vi "motor_outfeed_power.vi"(10 "Eject_Imp":dbl, 11 "Eject_Driver":dbl) -> (3 "Ele_Outfeed_Power_Power":dbl)   [LabVIEW 2014]
panel:
  in  "Outfeed Scalar [0,1]":dbl=1.0
  # "This is the motor outfeed power conversion"
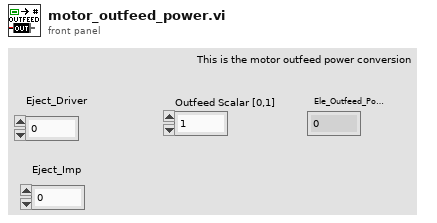
[diagram p1: front panel]
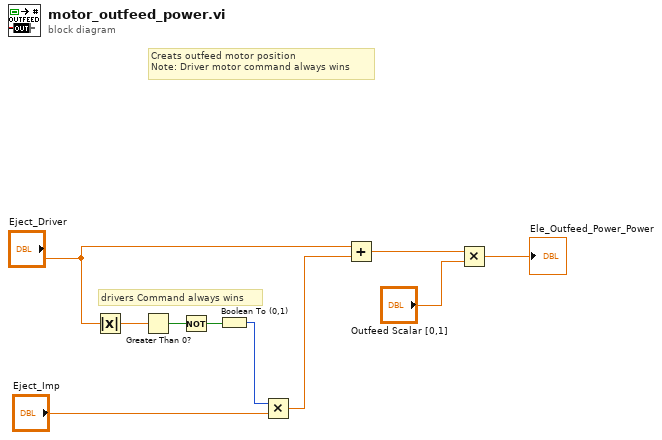
[diagram p0: block diagram]
diagram:
  # "drivers Command always wins"
  # "Creats outfeed motor position \nNote: Driver motor command always wins"
  n1 = Absolute Value(x="Eject_Driver") -> (abs(x)=w8:dbl)
  n2 = Greater Than 0?(x=w8) -> (x > 0?=w7:bool)
  n3 = Not(x=w7) -> (.not. x?=w5:bool)
  n4 = Boolean To (0,1)(Boolean=w5) -> (0, 1=w4:i16)
  n5 = Multiply(x=w4, y="Eject_Imp") -> (x*y=w1:dbl)
  n6 = Add(x="Eject_Driver", y=w1) -> (x+y=w3:dbl)
  n7 = Multiply(x=w3, y="Outfeed Scalar [0,1]") -> (x*y=→"Ele_Outfeed_Power_Power":dbl)
